vi "WSVCAP SHL FPGA LL RFFE Write Data.vi"(0 "CLK In":bool, 7 "Data Word In":u16, 11 "error in (no error)":errorcluster, 12 "Socket Mask":u16, 13 "Line":T1) -> (15 "error out":errorcluster)   [LabVIEW 2012]
uses:
  Type Defs/WSVCAP SHL RFFE Write Line Enum.ctl
  WSVCAP SHL FPGA LL RFFE Debug Global.vi
  <vilib>/eio/EIONode/EIONode.xnode
  <vilib>/rvi/eio/common/nirviEmuTemplateMethod_errors.vi
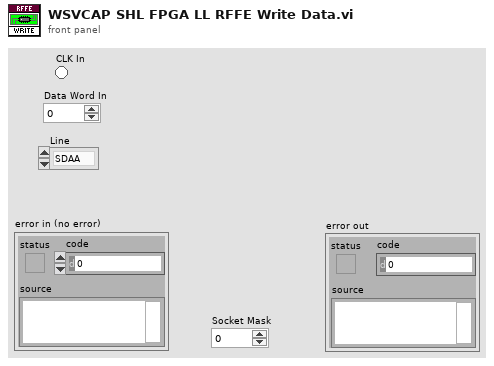
[diagram p1: front panel]
types:
  T1 = typedef "WSVCAP SHL RFFE Write Line Enum.ctl" = enum16{"SDAA", "SCLK"}
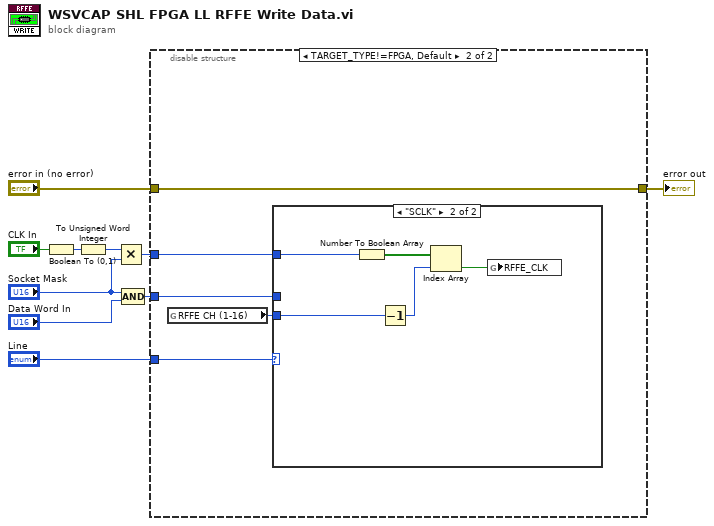
[diagram p0: block diagram]
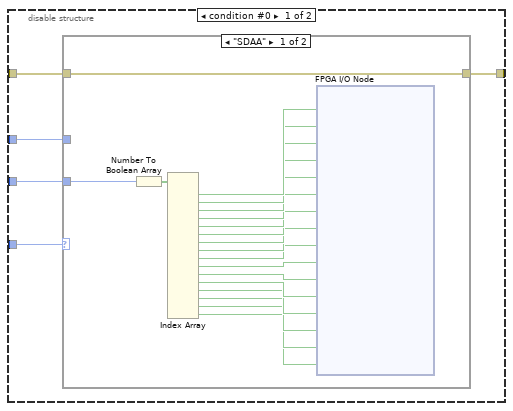
[diagram p2: hidden frame]
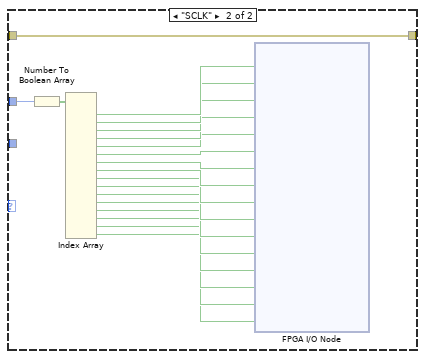
[diagram p3: hidden frame]
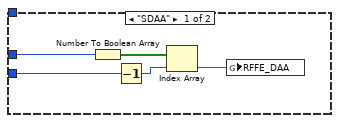
[diagram p4: hidden frame]
diagram:
  n1 = Boolean To (0,1)(Boolean="CLK In") -> (0, 1=w4:i16)
  n2 = To Unsigned Word Integer(number=w4) -> (unsigned 16bit integer=w3:u16)
  n3 = Multiply(x=w3, y="Socket Mask") -> (x*y=w1:u16)
  n4 = Compound Arithmetic op=AND("Socket Mask", "Data Word In") -> (w6:u16)
  n5 = disable-structure shown="TARGET_TYPE!=FPGA, Default" {
    disable-tunnel: "Line" -> [w15 w58]
    disable-tunnel: [w14 w57] -> w9
    disable-tunnel: "error in (no error)" -> [w13 w57]
    disable-tunnel: w6 -> [w12 w56]
    disable-tunnel: w1 -> [w11 w54]
    frame condition #0 {
      n6 = case shown="\"SDAA\"" w15 {
        tunnel: [w16 w35] -> w14
        tunnel: w13 -> [w16 w35]
        tunnel: w12 -> [w34 _]
        tunnel: w11 -> [_ w52]
        frame "SDAA" {
          n7 = Number To Boolean Array(number=w34) -> (Boolean array=w33:bool[])
          n8 = Index Array(array=w33) -> (element #1=w32:bool, element #2=w31:bool, element #3=w30:bool, element #4=w29:bool, element #5=w28:bool, element #6=w27:bool, element #7=w26:bool, element #8=w25:bool, element #9=w24:bool, element #10=w23:bool, element #11=w22:bool, element #12=w21:bool, element #13=w20:bool, element #14=w19:bool, element #15=w18:bool, element #16=w17:bool)  [unwired: 16 in]
          n9 = xnode "FPGA I/O Node"("RFFE_SDA_S1"=w32, "RFFE_SDA_S2"=w31, "RFFE_SDA_S3"=w30, "RFFE SDA_S4"=w29, "RFFE_SDA_S5"=w28, "RFFE_SDA_S6"=w27, "RFFE_SDA_S7"=w26, "RFFE_SDA_S8"=w25, "RFFE_SDA_S9"=w24, "RFFE_SDA_S10"=w23, "RFFE_SDA_S11"=w22, "RFFE_SDA_S12"=w21, "RFFE_SDA_S13"=w20, "RFFE_SDA_S14"=w19, "RFFE_SDA_S15"=w18, "RFFE_SDA_S16"=w17) -> ()  [unwired: 16 in, 16 out]
        }
        frame "SCLK" {
          n10 = Number To Boolean Array(number=w52) -> (Boolean array=w53:bool[])
          n11 = Index Array(array=w53) -> (element #1=w51:bool, element #2=w50:bool, element #3=w49:bool, element #4=w48:bool, element #5=w47:bool, element #6=w46:bool, element #7=w45:bool, element #8=w44:bool, element #9=w43:bool, element #10=w42:bool, element #11=w41:bool, element #12=w40:bool, element #13=w39:bool, element #14=w38:bool, element #15=w37:bool, element #16=w36:bool)  [unwired: 16 in]
          n12 = xnode "FPGA I/O Node"("RFFE_SCL_S1"=w51, "RFFE_SCL_S2"=w50, "RFFE_SCL_S3"=w49, "RFFE_SCL_S4"=w48, "RFFE_SCL_S5"=w47, "RFFE_SCL_S6"=w46, "RFFE_SCL_S7"=w45, "RFFE_SCL_S8"=w44, "RFFE_SCL_S9"=w43, "RFFE_SCL_S10"=w42, "RFFE_SCL_S11"=w41, "RFFE_SCL_S12"=w40, "RFFE_SCL_S13"=w39, "RFFE_SCL_S14"=w38, "RFFE_SCL_S15"=w37, "RFFE_SCL_S16"=w36) -> ()  [unwired: 16 in, 16 out]
        }
      }
    }
    frame condition #1 (active) {
      n13 = global read "WSVCAP SHL FPGA LL RFFE Debug Global.vi" "RFFE CH (1-16)"() -> (w55:i32)
      n14 = case shown="\"SCLK\"" w58 {
        tunnel: w56 -> [w60 _]
        tunnel: w55 -> [w59 w66]
        tunnel: w54 -> [_ w64]
        frame "SDAA" {
          n15 = Number To Boolean Array(number=w60) -> (Boolean array=w63:bool[])
          n16 = Decrement(x=w59) -> (x-1=w61:i32)
          n17 = Index Array(array=w63, index=w61) -> (element=w62:bool)
          n18 = global write "WSVCAP SHL FPGA LL RFFE Debug Global.vi" "RFFE_DAA"(w62) -> ()
        }
        frame "SCLK" {
          n19 = Number To Boolean Array(number=w64) -> (Boolean array=w68:bool[])
          n20 = Decrement(x=w66) -> (x-1=w67:i32)
          n21 = Index Array(array=w68, index=w67) -> (element=w65:bool)
          n22 = global write "WSVCAP SHL FPGA LL RFFE Debug Global.vi" "RFFE_CLK"(w65) -> ()
        }
      }
    }
  }
  "error out" <- w9
